vi "PerformOperation.vi"(1 "Operand 2":dbl, 2 "Operation":string(combo), 3 "Operand1":dbl) -> (0 "Answer":dbl)   [LabVIEW 2014]
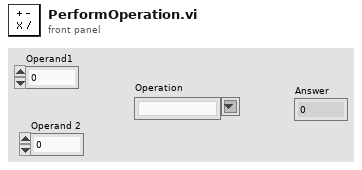
[diagram p1: front panel]
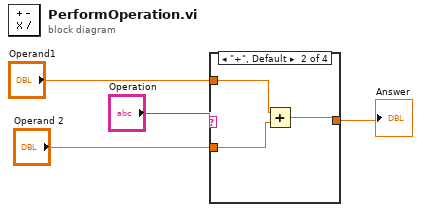
[diagram p0: block diagram]
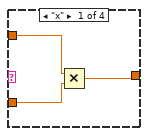
[diagram p2: hidden frame]
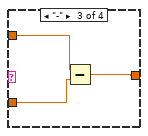
[diagram p3: hidden frame]
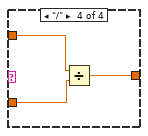
[diagram p4: hidden frame]
diagram:
  n1 = case shown="\"+\", Default" "Operation" {
    tunnel: "Operand1" -> [w7 w10 w13 w16]
    tunnel: "Operand 2" -> [w6 w9 w12 w15]
    tunnel: [w5 w8 w11 w14] -> w2
    frame "x" {
      n2 = Multiply(x=w7, y=w6) -> (x*y=w5:dbl)
    }
    frame "+", Default {
      n3 = Add(x=w10, y=w9) -> (x+y=w8:dbl)
    }
    frame "-" {
      n4 = Subtract(x=w13, y=w12) -> (x-y=w11:dbl)
    }
    frame "/" {
      n5 = Divide(x=w16, y=w15) -> (x/y=w14:dbl)
    }
  }
  "Answer" <- w2
